vi "Stop Core.vi"(10 "final error code":i32, 11 "Remote Operation Abstract in":refnum<class "Remote Operation Abstract.lvclass">) -> (3 "Remote Operation Abstract out":refnum<class "Remote Operation Abstract.lvclass">)   [LabVIEW 2018, in "Remote Operation Abstract.lvlib" / "Remote Operation Abstract.lvclass"]
doc: "(<B>Filename</B>: Actor Framework.lvlib:Actor.lvclass:Stop Core.vi)\n\nDefines what the actor does before it stops. Use the <B>final error code</B> input to determine whether the actor shut down in response to an error.\n\nBy default, this method does nothing. A descendant class may override it to define behavior, such as shutting down any processes the actor initiated in its override of the Actor Core method."
uses:
  Remote Operation Abstract.lvclass
  Remote Operation Abstract.lvclass/Remote Operation Abstract.ctl
  EMS Generic Actor/EMS Generic/EMS Generic.lvclass
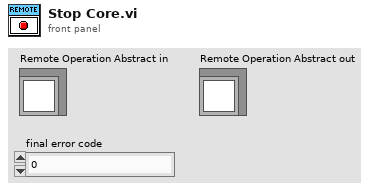
[diagram p1: front panel]
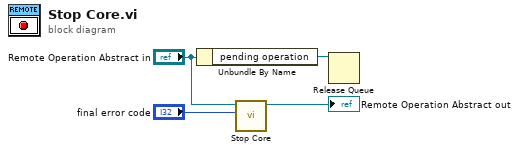
[diagram p0: block diagram]
diagram:
  n1 = Unbundle By Name("Remote Operation Abstract in") -> ("pending operation"=w1:refnum<queue>)
  n2 = call-parent "Stop Core.vi"("final error code"="final error code", "EMS Generic in"="Remote Operation Abstract in") -> ("EMS Generic out"=→"Remote Operation Abstract out":refnum<class "Remote Operation Abstract.lvclass">)  [unwired: 9 in]
  n3 = Release Queue(queue=w1) -> ()  [unwired: 2 in, 3 out]
